vi "_PC_Toolbar_Model_SetLayoutFloat.vi"(1 "MachineType":enum16{"None", "MALDI", "ESI"}(ring), 3 "ToolBar_Panel_Ref":refnum<vi>) -> (0 "TotalWidth":i32)   [LabVIEW 2018]
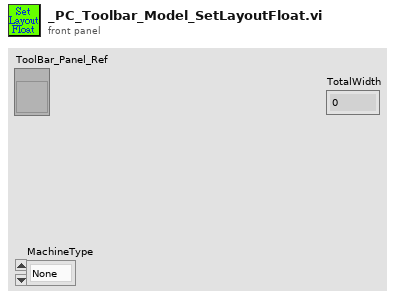
[diagram p1: front panel]
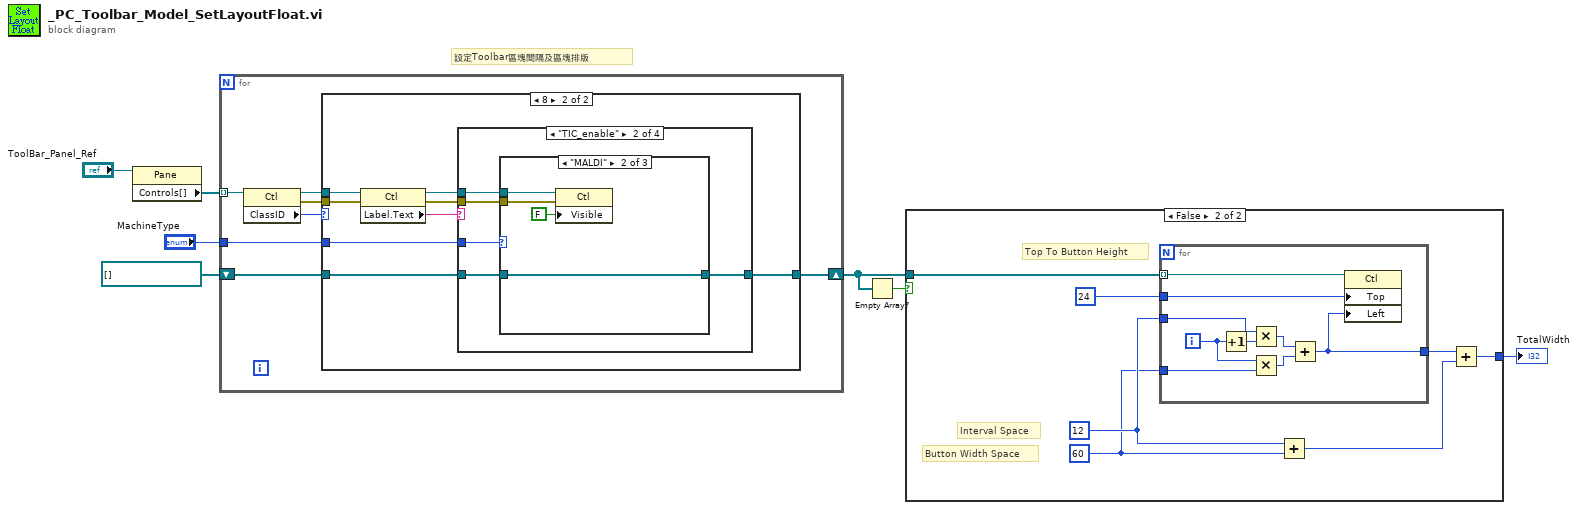
[diagram p0: block diagram]
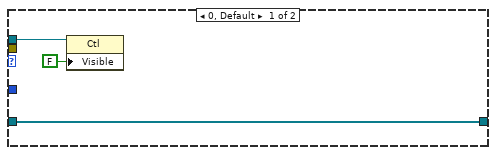
[diagram p2: hidden frame]
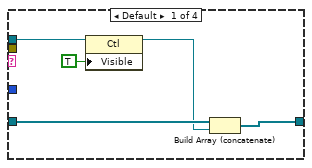
[diagram p3: hidden frame]
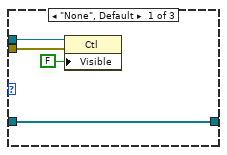
[diagram p4: hidden frame]
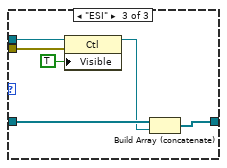
[diagram p5: hidden frame]
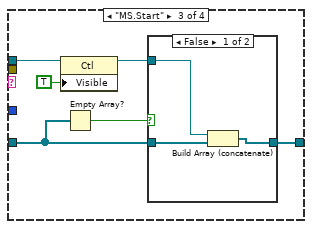
[diagram p6: hidden frame]
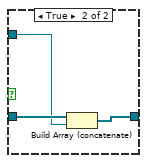
[diagram p7: hidden frame]
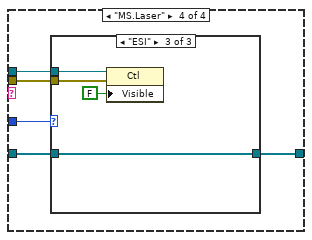
[diagram p8: hidden frame]
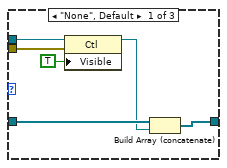
[diagram p9: hidden frame]
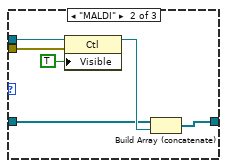
[diagram p10: hidden frame]
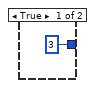
[diagram p11: hidden frame]
diagram:
  # "設定Toolbar區塊間隔及區塊排版"
  n1 = property class="Pane"(reference="ToolBar_Panel_Ref") -> ("Controls[]"=w5:refnum<vi>[])  [unwired: 1 in, 2 out]
  n2 = for {
    tunnel: w5 -> [w14] mode=indexing
    shift-right: [w9] -> w2
    shift-left: refnum<vi>[] [] -> [w13]
    tunnel: "MachineType" -> [w8]
    n3 = property class="Ctl"(reference=w14) -> (reference out=w11:refnum<vi>, error out=w10:errorcluster, "ClassID"=w12:u32)  [unwired: 1 in]
    n4 = case shown="8" w12 {
      tunnel: w11 -> [w17 w25]
      tunnel: w13 -> [w15 w20]
      tunnel: w10 -> [_ w24]
      tunnel: [w15 w19] -> w9
      tunnel: w8 -> [_ w18]
      frame 0, Default {
        n5 = property class="Ctl"(reference=w17, "Visible"=FALSE) -> ()  [unwired: 1 in, 2 out]
      }
      frame 8 {
        n6 = property class="Ctl"(reference=w25, error in=w24) -> (reference out=w22:refnum<vi>, error out=w21:errorcluster, "Label.Text"=w23:string)
        n7 = case shown="\"TIC_enable\"" w23 {
          tunnel: w22 -> [w28 w35 w55 w66]
          tunnel: w21 -> [_ w34 _ w65]
          tunnel: w20 -> [w30 w32 w51 w63]
          tunnel: [w29 w31 w50 w62] -> w19
          tunnel: w18 -> [_ w33 _ w64]
          frame Default {
            n8 = property class="Ctl"(reference=w28, "Visible"=TRUE) -> (reference out=w27:refnum<vi>)  [unwired: 1 in, 1 out]
            n9 = Build Array (concatenate)(w30, w27) -> (w29:refnum<vi>[])
          }
          frame "TIC_enable" {
            n10 = case shown="\"MALDI\"" w33 {
              tunnel: w35 -> [w38 w42 w48]
              tunnel: w34 -> [w37 w41 w47]
              tunnel: w32 -> [w36 w40 w46]
              tunnel: [w36 w40 w44] -> w31
              frame "None", Default {
                n11 = property class="Ctl"(reference=w38, error in=w37, "Visible"=FALSE) -> ()  [unwired: 2 out]
              }
              frame "MALDI" {
                n12 = property class="Ctl"(reference=w42, error in=w41, "Visible"=FALSE) -> ()  [unwired: 2 out]
              }
              frame "ESI" {
                n13 = property class="Ctl"(reference=w48, error in=w47, "Visible"=TRUE) -> (reference out=w45:refnum<vi>)  [unwired: 1 out]
                n14 = Build Array (concatenate)(w46, w45) -> (w44:refnum<vi>[])
              }
            }
          }
          frame "MS.Start" {
            n15 = property class="Ctl"(reference=w55, "Visible"=TRUE) -> (reference out=w52:refnum<vi>)  [unwired: 1 in, 1 out]
            n16 = Empty Array?(array=w51) -> (empty?=w53:bool)
            n17 = case shown="False" w53 {
              tunnel: w52 -> [w58 w60]
              tunnel: w51 -> [w57 w61]
              tunnel: [w56 w59] -> w50
              frame False {
                n18 = Build Array (concatenate)(w58, w57) -> (w56:refnum<vi>[])
              }
              frame True {
                n19 = Build Array (concatenate)(w61, w60) -> (w59:refnum<vi>[])
              }
            }
          }
          frame "MS.Laser" {
            n20 = case shown="\"ESI\"" w64 {
              tunnel: w66 -> [w71 w77 w81]
              tunnel: w65 -> [w70 w76 w80]
              tunnel: w63 -> [w69 w74 w79]
              tunnel: [w67 w73 w79] -> w62
              frame "None", Default {
                n21 = property class="Ctl"(reference=w71, error in=w70, "Visible"=TRUE) -> (reference out=w68:refnum<vi>)  [unwired: 1 out]
                n22 = Build Array (concatenate)(w69, w68) -> (w67:refnum<vi>[])
              }
              frame "MALDI" {
                n23 = property class="Ctl"(reference=w77, error in=w76, "Visible"=TRUE) -> (reference out=w75:refnum<vi>)  [unwired: 1 out]
                n24 = Build Array (concatenate)(w74, w75) -> (w73:refnum<vi>[])
              }
              frame "ESI" {
                n25 = property class="Ctl"(reference=w81, error in=w80, "Visible"=FALSE) -> ()  [unwired: 2 out]
              }
            }
          }
        }
      }
    }
  }
  n26 = Empty Array?(array=w2) -> (empty?=w1:bool)
  n27 = case shown="False" w1 {
    tunnel: [3 w86] -> w6
    tunnel: w2 -> [_ w84]
    frame True {
    }
    frame False {
      w88 = 60 ("y")
      w89 = 12 ("y")
      # "Button Width Space"
      # "Interval Space"
      # "Top To Button Height"
      n28 = for {
        tunnel: w84 -> [w91] mode=indexing
        tunnel: 24 ("Position:Top") -> [w99]
        tunnel: [w98] -> w90
        tunnel: w89 -> [w97]
        tunnel: w88 -> [w96]
        i -> [w95]
        n29 = Increment(x=w95) -> (x+1=w94:i32)
        n30 = Multiply(x=w97, y=w94) -> (x*y=w93:i32)
        n31 = Multiply(x=w95, y=w96) -> (x*y=w92:i32)
        n32 = Add(x=w93, y=w92) -> (x+y=w98:i32)
        n33 = property class="Ctl"(reference=w91, "Top"=w99, "Left"=w98) -> ()  [unwired: 1 in, 2 out]
      }
      n34 = Add(x=w89, y=w88) -> (x+y=w87:i32)
      n35 = Add(x=w90, y=w87) -> (x+y=w86:i32)
    }
  }
  "TotalWidth" <- w6
